vi "MVP02 Initialization VI.vi"(8 "error in (no error)":errorcluster, 10 "Custom XML":string, 11 "Device Item Ref in":T1 format="%.0x") -> (0 "error out":errorcluster, 3 "Device Item Ref out":T1 format="%.0x")   [LabVIEW 2016, in "MVP02 Custom Device.lvlib"]
uses:
  MVP02 Custom Device.lvlib
  <vilib>/NI Veristand/Custom Device API/Custom Device Item Ref.ctl
  <vilib>/NI Veristand/Custom Device API/Custom Device Channel.ctl
  <vilib>/NI Veristand/Custom Device API/Custom Device Channel Type.ctl
  <vilib>/NI Veristand/Custom Device API/Custom Device API.lvlib
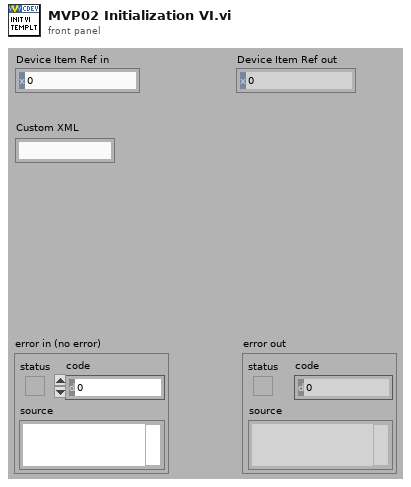
[diagram p1: front panel]
types:
  T1 = typedef "Custom Device API.lvlib/Custom Device Item Ref.ctl" = u64
  T2 = typedef "Custom Device API.lvlib/Custom Device Channel.ctl" = cluster{"Type":T3, "Units":string, "Default Value":dbl, "Faultable":bool, "Scalable":bool}
  T3 = typedef "Custom Device API.lvlib/Custom Device Channel Type.ctl" = enum16{"Input", "Output"}
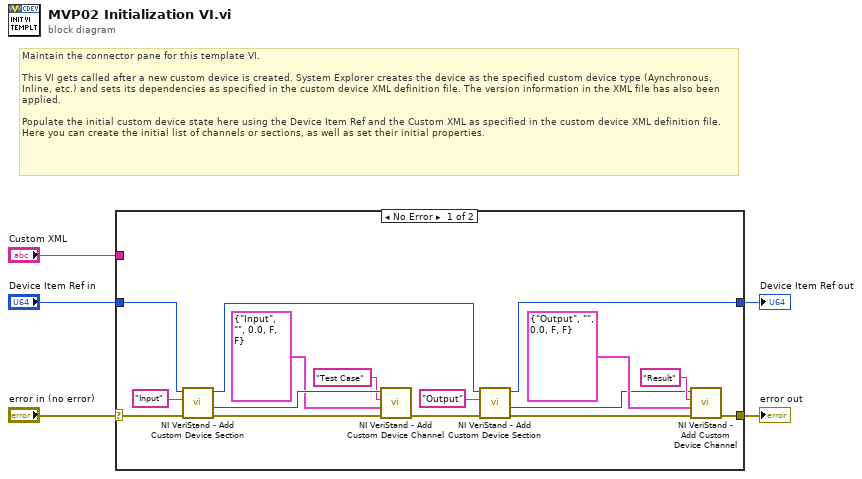
[diagram p0: block diagram]
diagram:
  # "Maintain the connector pane for this template VI.\n\nThis VI gets called after a new custom device is created. System Explorer creates the device as the specified custom device type (Aynchronous, Inline, etc.) and sets its dependencies as specified in the custom device XML definition file. The version information in the XML file has also been applied.\n\nPopulate the initial custom device state here using the Device Item Ref and the Custom XML as specified in the custom device XML definition file. Here you can create the initial list of channels or sections, as well as set their initial properties."
  n1 = case shown="No Error" "error in (no error)" {
    selector: "error in (no error)" -> [w20 w23]
    tunnel: [w9 w23] -> w5
    tunnel: [w8 w22] -> w3
    tunnel: "Device Item Ref in" -> [w7 w22]
    tunnel: "Custom XML" -> [_ _]
    frame No Error {
      n2 = call <vilib>:"NI VeriStand - Add Custom Device Section.vi"("error in (no error)"=w20, "Section Name"="Input", "Parent Ref in"=w7) -> ("error out"=w18:errorcluster, "Section Ptr"=w19:T1, "Parent Ref out"=w6:T1)  [unwired: 5 in, 1 out]
      n3 = call <vilib>:"NI VeriStand - Add Custom Device Channel.vi"("error in (no error)"=w18, "Channel"=T2 {"Type"=enum."Input", "Units"="", "Default Value"=0.0, "Faultable"=FALSE, "Scalable"=FALSE}, "Channel Name"="Test Case", "Parent Ref in"=w19) -> ("error out"=w10:errorcluster)  [unwired: 4 in, 3 out]
      n4 = call <vilib>:"NI VeriStand - Add Custom Device Section.vi"("error in (no error)"=w10, "Section Name"="Output", "Parent Ref in"=w6) -> ("error out"=w13:errorcluster, "Section Ptr"=w12:T1, "Parent Ref out"=w8:T1)  [unwired: 5 in, 1 out]
      n5 = call <vilib>:"NI VeriStand - Add Custom Device Channel.vi"("error in (no error)"=w13, "Channel"=T2 {"Type"=enum."Output", "Units"="", "Default Value"=0.0, "Faultable"=FALSE, "Scalable"=FALSE}, "Channel Name"="Result", "Parent Ref in"=w12) -> ("error out"=w9:errorcluster)  [unwired: 4 in, 3 out]
    }
    frame Error {
    }
  }
  "error out" <- w5
  "Device Item Ref out" <- w3
